vi "hj212-2017.vi"(0 "object in":refnum<class "212format_work.lvclass">, 1 "数据段":T1, 2 "PWD？":bool, 5 "error in (no error)":errorcluster) -> (14 "object out":refnum<class "212format_work.lvclass">, 15 "通讯包":T2={"包头（2）"="##", "数据段长度（4）"="", "数据段"="", "CRC校验"="", "包尾"=""}, 16 "通讯包字符串":string, 19 "error out":errorcluster)   [LabVIEW 2016, in "212format_work.lvclass"]
uses:
  212format_work.lvclass
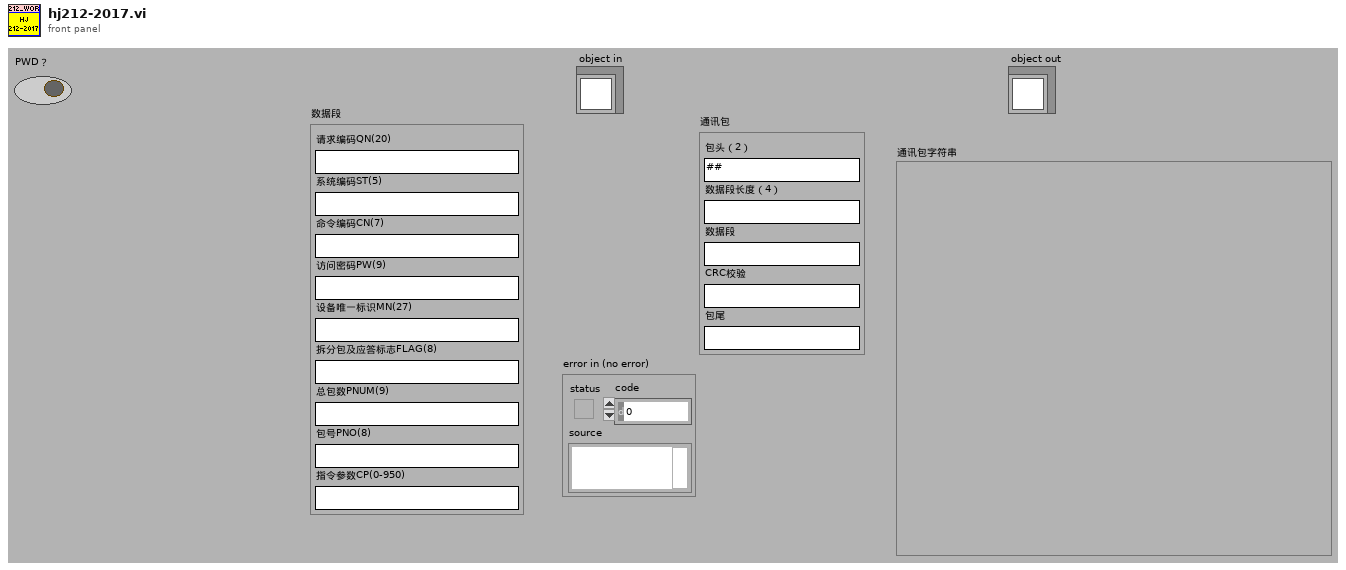
[diagram p1: front panel]
types:
  T1 = cluster{"请求编码QN(20)":string, "系统编码ST(5)":string, "命令编码CN(7)":string, "访问密码PW(9)":string, "设备唯一标识MN(27)":string, "拆分包及应答标志FLAG(8)":string, "总包数PNUM(9)":string, "包号PNO(8)":string, "指令参数CP(0-950)":string}
  T2 = cluster{"包头（2）":string, "数据段长度（4）":string, "数据段":string, "CRC校验":string, "包尾":string}
  T3 = typedef "212format_work.lvclass/interdata控件.ctl" = cluster{"数据发送协议":enum16{"2005-212协议", "2017-212协议"}, "枚举":enum16{"返回请求应答", "上传数据", "返回执行结果"}, "系统编码ST":string, "主动上报数据中":bool, "数据组合发送":bool, "地表水/污染源":bool, "应用环境":enum16{"STD", "GB212"}}
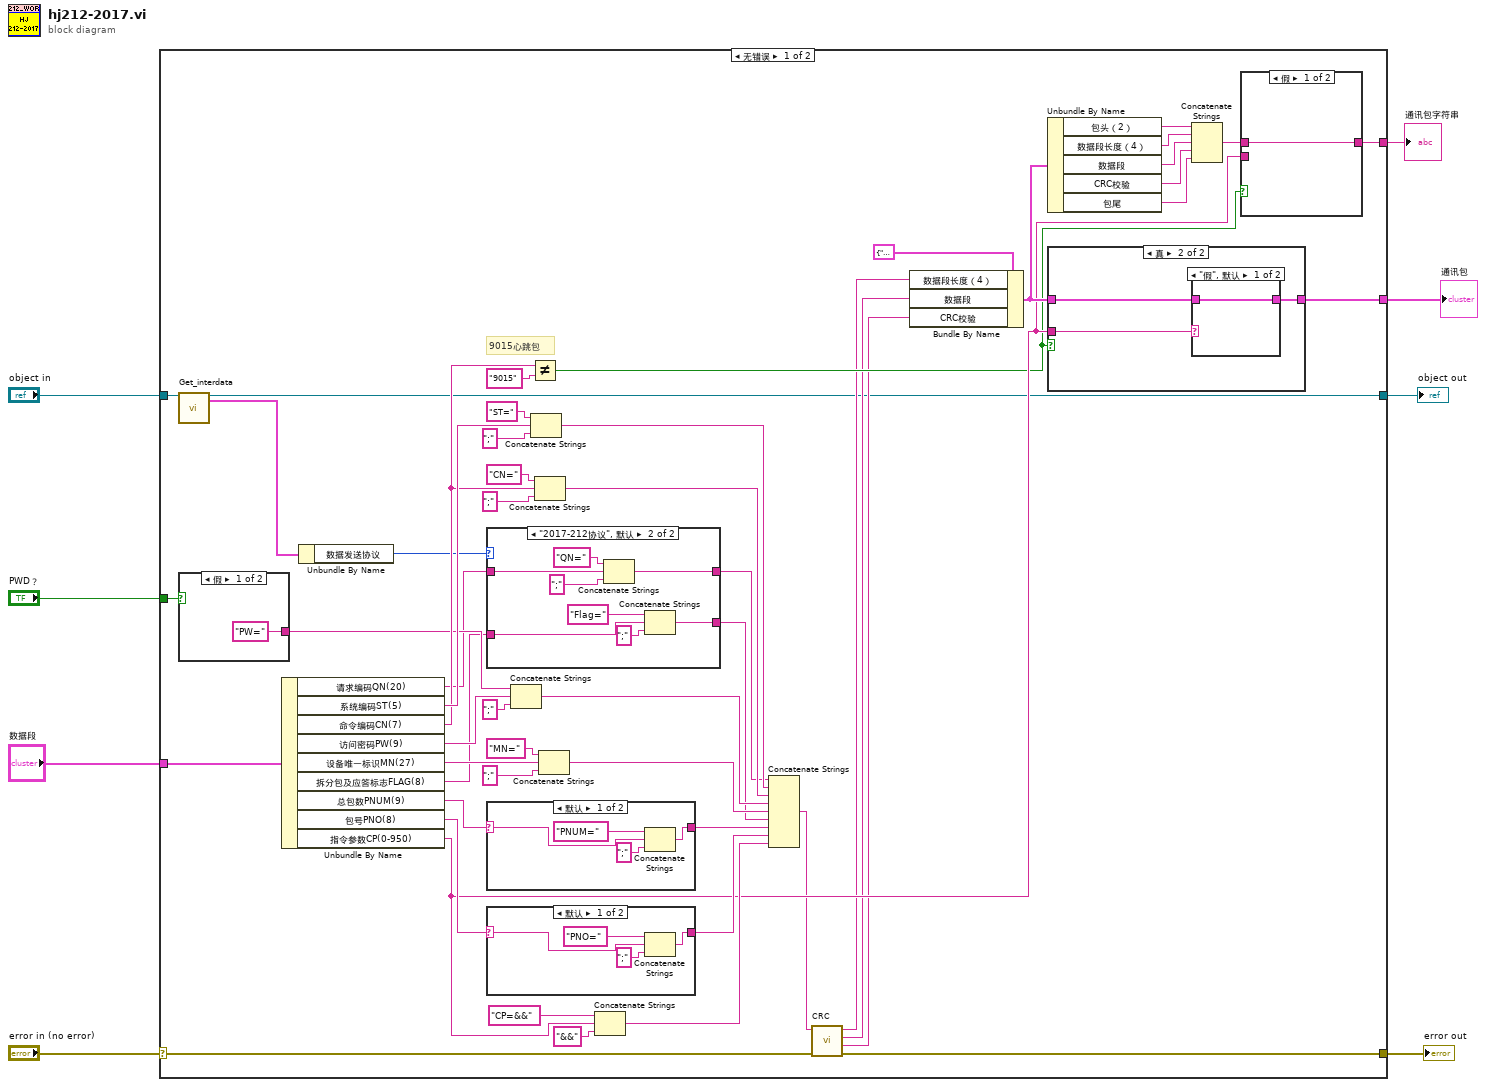
[diagram p0: block diagram]
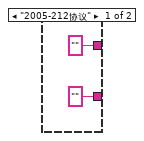
[diagram p2: hidden frame]
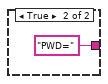
[diagram p3: hidden frame]
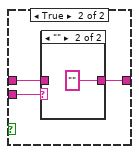
[diagram p4: hidden frame]
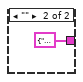
[diagram p7: hidden frame]
diagram:
  n1 = case shown="无错误" "error in (no error)" {
    selector: "error in (no error)" -> [w17 w96]
    tunnel: [w15 w96] -> w7
    tunnel: [w9 w95] -> w5
    tunnel: "object in" -> [w12 w95]
    tunnel: "数据段" -> [w22 _]
    tunnel: "PWD？" -> [w21 _]
    tunnel: [w20 _] -> w2
    tunnel: [w19 _] -> w1
    frame No Error {
      # "9015心跳包"
      n2 = call-dynamic "Get_interdata.vi"("object in"=w12) -> ("object out"=w9:refnum<class "212format_work.lvclass">, "interdata"=w11:T3)  [unwired: 16 in, 1 out]
      n3 = case shown="假" w21 {
        tunnel: ["PW=" ("字符串") "PWD=" ("字符串")] -> w27
        frame False {
        }
        frame True {
        }
      }
      n4 = Unbundle By Name(w22) -> ("请求编码QN(20)"=w26:string, "系统编码ST(5)"=w60:string, "命令编码CN(7)"=w30:string, "访问密码PW(9)"=w56:string, "设备唯一标识MN(27)"=w54:string, "拆分包及应答标志FLAG(8)"=w24:string, "总包数PNUM(9)"=w46:string, "包号PNO(8)"=w44:string, "指令参数CP(0-950)"=w31:string)
      n5 = Unbundle By Name(w11) -> ("数据发送协议"=w10:enum16{"2005-212协议", "2017-212协议"})
      n6 = case shown="\"2017-212协议\", 默认" w10 {
        tunnel: w26 -> [_ w66]
        tunnel: ["" w65] -> w25
        tunnel: w24 -> [_ w64]
        tunnel: ["" w63] -> w23
        frame "2005-212协议" {
        }
        frame "2017-212协议", Default {
          n7 = Concatenate Strings("QN=" ("字符串"), w66, ";" ("字符串")) -> (w65:string)
          n8 = Concatenate Strings("Flag=" ("字符串"), w64, ";" ("字符串")) -> (w63:string)
        }
      }
      n9 = case shown="默认" w46 {
        selector: w46 -> [w92 w94]
        tunnel: [w90 w94] -> w45
        frame Default {
          n10 = Concatenate Strings("PNUM=" ("字符串"), w92, ";" ("字符串")) -> (w90:string)
        }
        frame "" {
        }
      }
      n11 = case shown="默认" w44 {
        selector: w44 -> [w87 w89]
        tunnel: [w85 w89] -> w43
        frame Default {
          n12 = Concatenate Strings("PNO=" ("字符串"), w87, ";" ("字符串")) -> (w85:string)
        }
        frame "" {
        }
      }
      n13 = Concatenate Strings(w27, w56, ";" ("字符串")) -> (w49:string)
      n14 = Not Equal?(x=w30, y="9015") -> (x != y?=w28:bool)
      n15 = Concatenate Strings("ST=" ("字符串"), w60, ";" ("字符串")) -> (w51:string)
      n16 = Concatenate Strings("CN=" ("字符串"), w30, ";" ("字符串")) -> (w50:string)
      n17 = Concatenate Strings("MN=" ("字符串"), w54, ";" ("字符串")) -> (w48:string)
      n18 = Concatenate Strings("CP=&&" ("字符串"), w31, "&&" ("字符串")) -> (w40:string)
      n19 = Concatenate Strings(w25, w51, w50, w49, w48, w23, w45, w43, w40) -> (w18:string)
      n20 = call "CRC.vi"("error in (no error)"=w17, "puchMsg"=w18) -> ("error out"=w15:errorcluster, "CRC校验"=w13:string, "数据段"=w14:string, "数据段长度"=w16:string)  [unwired: 6 in]
      n21 = Bundle By Name(cluster=T2 {"包头（2）"="##", "数据段长度（4）"="", "数据段"="", "CRC校验"="", "包尾"="\r\n"} ("通讯包"), "数据段长度（4）"=w16, "数据段"=w14, "CRC校验"=w13) -> (w32:T2)
      n22 = Unbundle By Name(w32) -> ("包头（2）"=w38:string, "数据段长度（4）"=w37:string, "数据段"=w36:string, "CRC校验"=w35:string, "包尾"=w34:string)
      n23 = case shown="真" w28 {
        tunnel: w32 -> [w79 w82]
        tunnel: [w79 w81] -> w19
        tunnel: w31 -> [_ w80]
        frame False {
        }
        frame True {
          n24 = case shown="\"假\", 默认" w80 {
            tunnel: [w83 T2 {"包头（2）"="", "数据段长度（4）"="", "数据段"="", "CRC校验"="", "包尾"=""} ("通讯包")] -> w81
            tunnel: w82 -> [w83 _]
            frame "假", Default {
            }
            frame "" {
            }
          }
        }
      }
      n25 = Concatenate Strings(w38, w37, w36, w35, w34) -> (w33:string)
      n26 = case shown="假" w28 {
        tunnel: w33 -> [w73 w76]
        tunnel: [w73 w75] -> w20
        tunnel: w31 -> [_ w74]
        frame False {
        }
        frame True {
          n27 = case shown="\"\"" w74 {
            tunnel: [w77 ""] -> w75
            tunnel: w76 -> [w77 _]
            frame "假", Default {
            }
            frame "" {
            }
          }
        }
      }
    }
    frame Error {
    }
  }
  "error out" <- w7
  "object out" <- w5
  "通讯包" <- w1
  "通讯包字符串" <- w2
